vi "IMS Stepper Move Scaled.vi"() -> ()   [LabVIEW 2017]
panel:
  in  "Scale Factor":dbl=-47.2441
  out "Position":dbl format="%.4f"
  out "error out":errorcluster
  in  "Mode":bool
  in  "Distance":dbl=1.0 min=-193273528.32 max=193273528.0 format="%.2f"
  in  "Instrument Address":refnum<visa-resource-name>
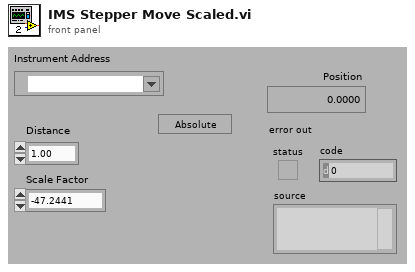
[diagram p1: front panel]
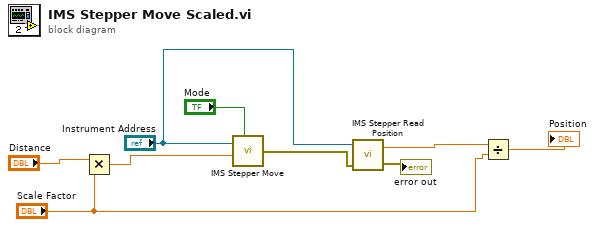
[diagram p0: block diagram]
diagram:
  n1 = Multiply(x="Distance", y="Scale Factor") -> (x*y=w3:dbl)
  n2 = call "IMS Stepper Move.vi"("Instrument Address"="Instrument Address", "Distance"=w3, "Mode"="Mode") -> ("error out"=w7:errorcluster)  [unwired: 2 in]
  n3 = call "IMS Stepper Read Position.vi"("error in (no error)"=w7, "Instrument Address"="Instrument Address") -> ("error out"=→"error out":errorcluster, "Response"=w4:dbl)  [unwired: 1 in]
  n4 = Divide(x=w4, y="Scale Factor") -> (x/y=→"Position":dbl)
